vi "Send status.vi"(8 "error in (no error)":errorcluster, 11 "Channel in":refnum<class "SPARC4_Channel.lvclass">) -> (0 "error out":errorcluster, 3 "Channel out":refnum<class "SPARC4_Channel.lvclass">)   [LabVIEW 2018, in "SPARC4_Channel.lvclass"]
uses:
  SPARC4_Channel.lvclass
  C:/Users/Denis/Desktop/S4ACS/S4ACS/Channel/Channel.lvclass
  SPARC4_Channel.lvclass/SPARC4_Channel.ctl
  Server/Server.lvclass/Server.ctl
  Sim_CCD/Sim_CCD.lvclass/Sim_CCD.ctl
  RxTx/RxTx.lvclass
  Sim_CCD/Sim_CCD.lvclass
  Server/Server.lvclass
  Channel/Channel.lvclass
panel:
  in  "status message":T1
  in  "Camera Status":T2
  in  "comm status":T3
  in  "Prev SET parameters":T4
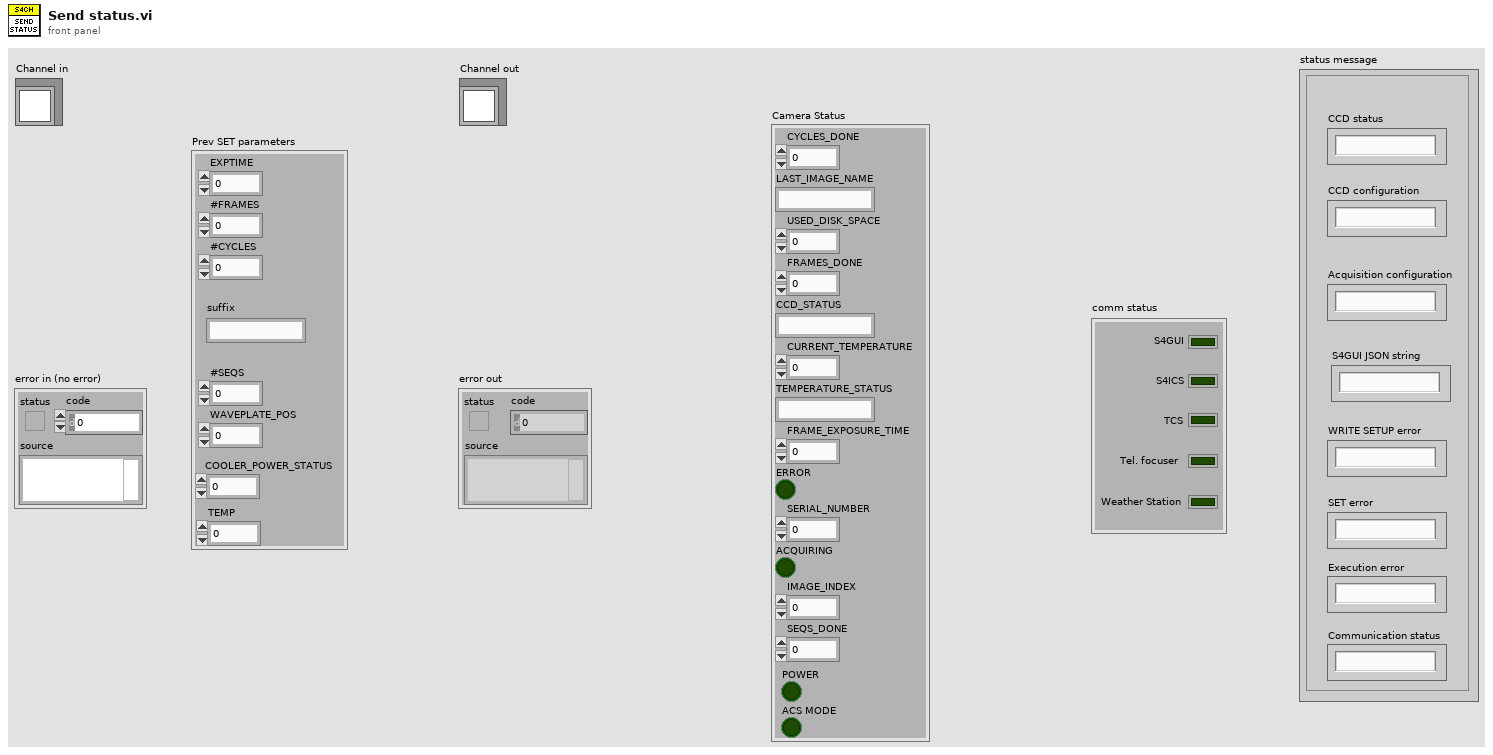
[diagram p1: front panel]
types:
  T1 = cluster{"CCD status":string, "CCD configuration":string, "Acquisition configuration":string, "S4GUI JSON string":string, "WRITE SETUP error":string, "Execution error":string, "SET error":string, "Communication status":string}
  T2 = cluster{"CYCLES_DONE":u16, "LAST_IMAGE_NAME":string, "USED_DISK_SPACE":u16, "FRAMES_DONE":u16, "CCD_STATUS":string, "CURRENT_TEMPERATURE":i16, "TEMPERATURE_STATUS":string, "FRAME_EXPOSURE_TIME":sgl, "ERROR":bool, "SERIAL_NUMBER":u16, "ACQUIRING":bool, "IMAGE_INDEX":u32, "SEQS_DONE":u16, "POWER":bool, "ACS MODE":bool}
  T3 = cluster{"S4GUI":bool, "S4ICS":bool, "TCS":bool, "Weather Station":bool, "Tel. focuser":bool}
  T4 = cluster{"EXPTIME":dbl, "#FRAMES":u32, "#CYCLES":u32, "#SEQS":u32, "WAVEPLATE_POS":u16, "suffix":string, "COOLER_POWER_STATUS":u8, "TEMP":i32}
  T5 = cluster{"CYCLES_DONE":u16, "LAST_IMAGE_NAME":string, "USED_DISK_SPACE":u16, "IMAGE_INDEX":u32, "acquisition error":bool}
  T6 = cluster{"SEQS_DONE":u16, "S4ICS comm attempts":u8}
  T7 = cluster{"State Machine.lvclass":refnum<class "State Machine.lvclass">, "RxTx.lvclass":refnum<class "RxTx.lvclass">, "Save_Header_RxTx.lvclass":refnum<class "RxTx.lvclass">, "Status SM.lvclass":refnum<class "State Machine.lvclass">, "Status RxTx.lvclass":refnum<class "RxTx.lvclass">, "servers array":refnum<class "Server.lvclass">[], "Events log file.lvclass":refnum<class "Log File.lvclass">, "Errors log file.lvclass":refnum<class "Log File.lvclass">, "Keywords log file.lvclass":refnum<class "Log File.lvclass">, "Sim_CCD.lvclass":refnum<class "Sim_CCD.lvclass">}
  T8 = cluster{"FRAMES_DONE":u16, "CCD_STATUS":string, "CURRENT_TEMPERATURE":i16, "TEMPERATURE_STATUS":string, "FRAME_EXPOSURE_TIME":sgl, "SERIAL_NUMBER":u16, "ACQUIRING":bool, "POWER":bool, "ACS MODE":bool}
  T9 = cluster{"PREAMP":u16, "READOUT_RATE":u16, "VERTICAL_SHIFT_SPEED":u16, "READ_MODE":u16, "VERTICAL_CLOCK_VOLTAGE":u16, "ACQUISITION_MODE":u16, "AD_CHANNEL":u16, "SHUTTER_TTL":u16, "SHUTTER_OPENING_TIME":u16, "SHUTTER_CLOSING_TIME":u16, "SHUTTER_MODE":u16, "TRIGGER_MODE":u16, "VBIN":u16, "INITIAL_LINE":u16, "INITIAL_COLUMN":u16, "FINAL_LINE":u16, "FINAL_COLUMN":u16, "HBIN":u16}
  T10 = cluster{"EXPTIME":dbl, "#FRAMES":u32, "COOLER_POWER_STATUS":u16, "TEMP":i32}
  T11 = cluster{"EXPTIME":errorcluster, "#FRAMES":errorcluster, "COOLER_POWER_STATUS":errorcluster, "TEMP":errorcluster}
  T12 = cluster{"CCD status":string, "camera op mode":string, "acq config":string, "GUI status msg":string, "op mode errors":string, "acq config error":string, "comm status":string}
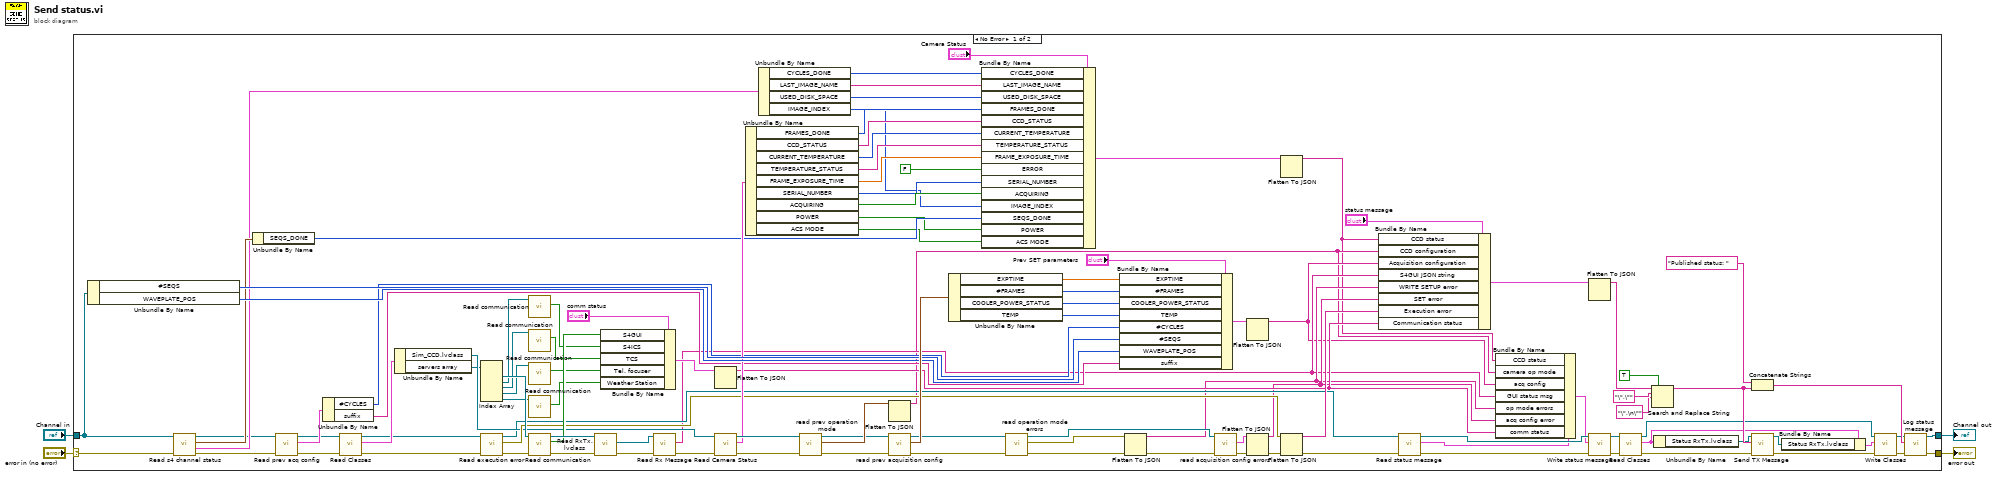
[diagram p0: block diagram]
diagram:
  n1 = case shown="No Error" "error in (no error)" {
    selector: "error in (no error)" -> [w36 w118]
    tunnel: [w72 w118] -> w3
    tunnel: [w71 w117] -> w1
    tunnel: "Channel in" -> [w35 w117]
    frame No Error {
      n2 = Unbundle By Name(w35) -> ("#SEQS"=w67:u32, "WAVEPLATE_POS"=w66:i32)
      n3 = call "Read s4 channel status.vi"("error in (no error)"=w36, "SPARC4_Channel in"=w35) -> ("error out"=w38:errorcluster, "channel status"=w48:T5, "s4 channel status"=w50:T6, "SPARC4_Channel out"=w37:refnum<class "SPARC4_Channel.lvclass">)  [unwired: 6 in]
      n4 = Unbundle By Name(w50) -> ("SEQS_DONE"=w49:u16)
      n5 = call-dynamic "Read prev acq config.vi"("error in (no error)"=w38, "Channel in"=w37) -> ("error out"=w40:errorcluster, "prev acq config"=w47:cluster{"suffix":string, "#CYCLES":u32}, "Channel out"=w39:refnum<class "SPARC4_Channel.lvclass">)  [unwired: 7 in]
      n6 = Unbundle By Name(w47) -> ("#CYCLES"=w45:u32, "suffix"=w46:string)
      n7 = call-dynamic "Read Classes.vi"("error in (no error)"=w40, "Channel in"=w39) -> ("error out"=w33:errorcluster, "Classes"=w43:T7, "Channel out"=w34:refnum<class "SPARC4_Channel.lvclass">)  [unwired: 7 in]
      n8 = Unbundle By Name(w43) -> ("Sim_CCD.lvclass"=w42:refnum<class "Sim_CCD.lvclass">, "servers array"=w41:refnum<class "Server.lvclass">[])
      n9 = Index Array(array=w41) -> (element #1=w86:refnum<class "Server.lvclass">, element #2=w83:refnum<class "Server.lvclass">, element #3=w82:refnum<class "Server.lvclass">, element #4=w81:refnum<class "Server.lvclass">, element #5=w80:refnum<class "Server.lvclass">)  [unwired: 5 in]
      n10 = call-dynamic "Read execution error.vi"("error in (no error)"=w33, "Channel in"=w34) -> ("error out"=w32:errorcluster, "execution error"=w44:errorcluster, "Channel out"=w31:refnum<class "SPARC4_Channel.lvclass">)  [unwired: 7 in]
      n11 = call "Read communication.vi"("Server in"=w83) -> ("communication"=w77:bool)  [unwired: 8 in, 2 out]
      n12 = call "Read communication.vi"("Server in"=w82) -> ("communication"=w76:bool)  [unwired: 8 in, 2 out]
      n13 = call "Read communication.vi"("Server in"=w81) -> ("communication"=w75:bool)  [unwired: 8 in, 2 out]
      n14 = call "Read communication.vi"("Server in"=w80) -> ("communication"=w74:bool)  [unwired: 8 in, 2 out]
      n15 = call "Read communication.vi"("error in (no error)"=w32, "Server in"=w86) -> ("error out"=w84:errorcluster, "communication"=w78:bool, "Server out"=w85:refnum<class "Server.lvclass">)  [unwired: 7 in]
      n16 = call "Read RxTx.lvclass.vi"("error in (no error)"=w84, "Server in"=w85) -> ("error out"=w101:errorcluster, "RxTx.lvclass"=w102:refnum<class "RxTx.lvclass">)  [unwired: 7 in, 1 out]
      n17 = Bundle By Name(cluster="comm status", "S4GUI"=w78, "S4ICS"=w77, "TCS"=w76, "Tel. focuser"=w75, "Weather Station"=w74) -> (w73:T3)
      n18 = call "Read Rx Message.vi"("error in (no error)"=w101, "RxTx in"=w102) -> ("error out"=w100:errorcluster, "Rx Message"=w12:string)  [unwired: 7 in, 1 out]
      n19 = Flatten To JSON(anything=w73) -> (JSON string=w15:string)  [unwired: 2 in, 1 out]
      n20 = call "Read Camera Status.vi"("error in (no error)"=w100, "CCDCamera in"=w42) -> ("error out"=w114:errorcluster, "camera status"=w63:T8, "CCDCamera out"=w115:refnum<class "Sim_CCD.lvclass">)  [unwired: 7 in]
      n21 = Unbundle By Name(w63) -> ("FRAMES_DONE"=w56:u16, "CCD_STATUS"=w57:string, "CURRENT_TEMPERATURE"=w58:i16, "TEMPERATURE_STATUS"=w59:string, "FRAME_EXPOSURE_TIME"=w60:sgl, "SERIAL_NUMBER"=w61:u16, "ACQUIRING"=w62:bool, "POWER"=w8:bool, "ACS MODE"=w7:bool)
      n22 = Unbundle By Name(w48) -> ("CYCLES_DONE"=w55:u16, "LAST_IMAGE_NAME"=w54:string, "USED_DISK_SPACE"=w53:u16, "IMAGE_INDEX"=w52:u32)
      n23 = call "read prev operation mode.vi"("error in (no error)"=w114, "Simulated_CCD_Camera in"=w115) -> ("error out"=w112:errorcluster, "prev operation mode"=w116:T9, "Simulated_CCD_Camera out"=w113:refnum<class "Sim_CCD.lvclass">)  [unwired: 7 in]
      n24 = Flatten To JSON(anything=w116) -> (JSON string=w10:string)  [unwired: 2 in, 1 out]
      n25 = call "read prev acquisition config.vi"("error in (no error)"=w112, "Simulated_CCD_Camera in"=w113) -> ("error out"=w97:errorcluster, "prev acquisition configuration"=w105:T10, "Simulated_CCD_Camera out"=w95:refnum<class "Sim_CCD.lvclass">)  [unwired: 7 in]
      n26 = Unbundle By Name(w105) -> ("EXPTIME"=w104:dbl, "#FRAMES"=w103:u32, "COOLER_POWER_STATUS"=w5:u16, "TEMP"=w6:i32)
      n27 = Bundle By Name(cluster="Camera Status", "CYCLES_DONE"=w55, "LAST_IMAGE_NAME"=w54, "USED_DISK_SPACE"=w53, "FRAMES_DONE"=w56, "CCD_STATUS"=w57, "CURRENT_TEMPERATURE"=w58, "TEMPERATURE_STATUS"=w59, "FRAME_EXPOSURE_TIME"=w60, "ERROR"=FALSE, "SERIAL_NUMBER"=w61, "ACQUIRING"=w62, "IMAGE_INDEX"=w52, "SEQS_DONE"=w49, "POWER"=w8, "ACS MODE"=w7) -> (w64:T2)
      n28 = call "read operation mode errors.vi"("error in (no error)"=w97, "Simulated_CCD_Camera in"=w95) -> ("error out"=w90:errorcluster, "WRITE SETUP errors"=w91:errorcluster[], "Simulated_CCD_Camera out"=w96:refnum<class "Sim_CCD.lvclass">)  [unwired: 7 in]
      n29 = Bundle By Name(cluster="Prev SET parameters", "EXPTIME"=w104, "#FRAMES"=w103, "COOLER_POWER_STATUS"=w5, "TEMP"=w6, "#CYCLES"=w45, "#SEQS"=w67, "WAVEPLATE_POS"=w66, "suffix"=w46) -> (w106:T4)
      n30 = Flatten To JSON(anything=w91, error in (no error)=w90) -> (JSON string=w13:string, 11:w89:errorcluster)  [unwired: 1 in]
      n31 = call "read acquisition config errors.vi"("error in (no error)"=w89, "Simulated Camera in"=w96) -> ("error out"=w94:errorcluster, "acquisition config errors"=w88:T11)  [unwired: 7 in, 1 out]
      n32 = Flatten To JSON(anything=w106) -> (JSON string=w11:string)  [unwired: 2 in, 1 out]
      n33 = Flatten To JSON(anything=w88, error in (no error)=w94) -> (JSON string=w14:string, 11:w93:errorcluster)  [unwired: 1 in]
      n34 = Flatten To JSON(anything=w64) -> (JSON string=w9:string)  [unwired: 2 in, 1 out]
      n35 = Flatten To JSON(anything=w44, error in (no error)=w93) -> (JSON string=w87:string, 11:w92:errorcluster)  [unwired: 1 in]
      n36 = Bundle By Name(cluster="status message", "CCD status"=w9, "CCD configuration"=w10, "Acquisition configuration"=w11, "S4GUI JSON string"=w12, "WRITE SETUP error"=w13, "SET error"=w14, "Execution error"=w87, "Communication status"=w15) -> (w16:T1)
      n37 = call "Read status message.vi"("error in (no error)"=w92, "Channel in"=w31) -> ("error out"=w98:errorcluster, "status message"=w18:T12, "Channel out"=w99:refnum<class "SPARC4_Channel.lvclass">)  [unwired: 7 in]
      n38 = Bundle By Name(cluster=w18, "CCD status"=w9, "camera op mode"=w10, "acq config"=w11, "GUI status msg"=w12, "op mode errors"=w13, "acq config error"=w14, "comm status"=w15) -> (w17:T12)
      n39 = Flatten To JSON(anything=w16) -> (JSON string=w111:string)  [unwired: 2 in, 1 out]
      n40 = call "Write status message.vi"("error in (no error)"=w98, "status message"=w17, "Channel in"=w99) -> ("error out"=w28:errorcluster, "Channel out"=w27:refnum<class "SPARC4_Channel.lvclass">)  [unwired: 7 in]
      n41 = call-dynamic "Read Classes.vi"("error in (no error)"=w28, "Channel in"=w27) -> ("error out"=w25:errorcluster, "Classes"=w24:T7, "Channel out"=w22:refnum<class "SPARC4_Channel.lvclass">)  [unwired: 7 in]
      n42 = Search and Replace String(replace all?=TRUE ("replace all? (F)"), input string=w111, search string="\",\"", replace string="\",\n\"" ("search string")) -> (result string=w70:string)  [unwired: 4 in, 3 out]
      n43 = Unbundle By Name(w24) -> ("Status RxTx.lvclass"=w26:refnum<class "RxTx.lvclass">)
      n44 = Concatenate Strings("Published status: " ("string"), w70) -> (w69:string)
      n45 = call "Send TX Message.vi"("error in (no error)"=w25, "message"=w70, "RxTx in"=w26) -> ("error out"=w21:errorcluster, "RxTx out"=w20:refnum<class "RxTx.lvclass">)  [unwired: 7 in]
      n46 = Bundle By Name(cluster=w24, "Status RxTx.lvclass"=w20) -> (w23:T7)
      n47 = call-dynamic "Write Classes.vi"("error in (no error)"=w21, "Classes"=w23, "Channel in"=w22) -> ("error out"=w30:errorcluster, "Channel out"=w29:refnum<class "SPARC4_Channel.lvclass">)  [unwired: 7 in]
      n48 = call "Log status message.vi"("error in (no error)"=w30, "String"=w69, "Channel in"=w29) -> ("error out"=w72:errorcluster, "Channel out"=w71:refnum<class "SPARC4_Channel.lvclass">)  [unwired: 7 in]
    }
    frame Error {
    }
  }
  "error out" <- w3
  "Channel out" <- w1
